vi "add tags for channels.vi"(5 "outputs?":bool[](array[boolean]), 7 "module instance":string, 8 "create input tags?":bool, 9 "create output tags?":bool, 10 "channels":refnum<class "EIP Tags Channel.lvclass">[](array[class]), 11 "engine configuration in":refnum<class "engine configuration.lvclass">) -> (0 "error IO":errorcluster, 3 "engine configuration out":refnum<class "engine configuration.lvclass">)   [LabVIEW 2013, in "EIP Tags editor node.lvclass"]
uses:
  EIP Tags editor node.lvclass
  <vilib>/NI/Module Execution Interface/Engine Configuration/engine configuration.lvclass
  channel/EIP Tags Channel.lvclass
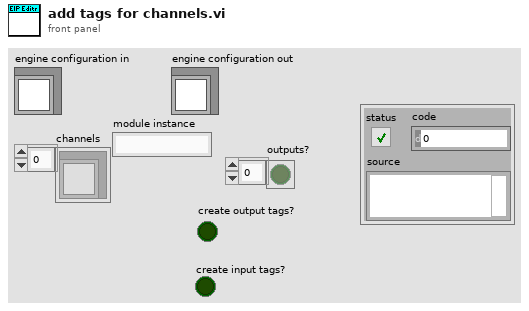
[diagram p1: front panel]
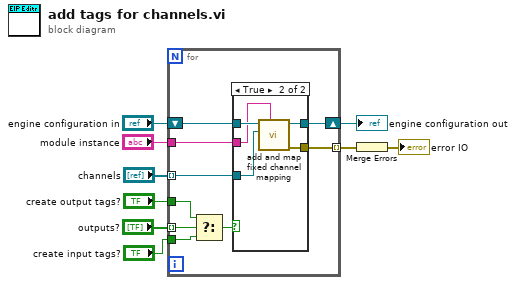
[diagram p0: block diagram]
diagram:
  n1 = for {
    tunnel: "channels" -> [w16] mode=indexing
    shift-right: [w17] -> w8
    shift-left: "engine configuration in" -> [w18]
    tunnel: [w15] -> w5 mode=indexing
    tunnel: "module instance" -> [w14]
    tunnel: "outputs?" -> [w13] mode=indexing
    tunnel: "create output tags?" -> [w12]
    tunnel: "create input tags?" -> [w11]
    n2 = Select(t=w12, s=w13, f=w11) -> (s? t:f=w10:bool)
    n3 = case shown="True" w10 {
      tunnel: w18 -> [w19 w24]
      tunnel: [w19 w23] -> w17
      tunnel: w16 -> [_ w22]
      tunnel: [_ w21] -> w15
      tunnel: w14 -> [_ w20]
      frame False {
      }
      frame True {
        n4 = call <vilib>:"add and map fixed channel mapping.vi"("module instance"=w20, "fixed channel"=w22, "engine configuration in"=w24) -> ("error out"=w21:errorcluster, "engine configuration out"=w23:refnum<class "engine configuration.lvclass">)  [unwired: 7 in]
      }
    }
  }
  "engine configuration out" <- w8
  n5 = Merge Errors(w5) -> (→"error IO":errorcluster)
